vi "drawConnectionArrow.vi"(0 "reference":refnum<class "Graphics.lvclass">, 1 "point2D":T1 {"y" format="%.2f"; "x" format="%.2f"}, 3 "color(if not used=default color)":u32=536870912 format="%.0x", 4 "fill?(F)":bool, 5 "error in (no error)":errorcluster, 6 "Label":string, 8 "Can'tGoLeft":bool) -> (14 "reference out":refnum<class "Graphics.lvclass">, 19 "error out":errorcluster)   [LabVIEW 2016, in "Graphics.lvclass"]
uses:
  <resource>/Framework/Providers/Open_GDS/UML/Graphics_class/Graphics.lvclass
  <resource>/Framework/Providers/Open_GDS/UML/General/Point/Point Point2D.ctl
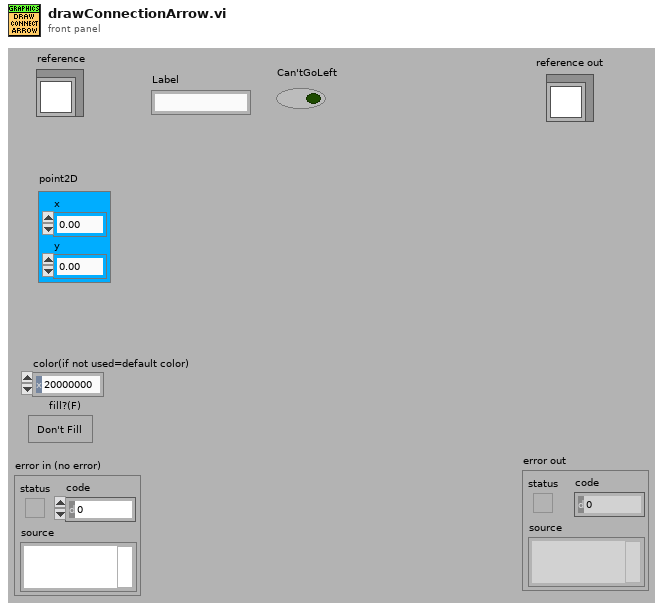
[diagram p1: front panel]
types:
  T1 = typedef "Point Point2D.ctl" = cluster{"x":dbl, "y":dbl}
  T2 = cluster{"horizontal":enum16{"left", "center", "right"}, "vertical":enum16{"top", "center", "bottom"}}
  T3 = typedef "Graphics.lvclass/ObjectAttributes.ctl" = cluster{"drawColor":u32, "backgroundColor":u32, "font":T4, "fontType":T5, "picture":picture, "stroke":T6, "scaleX":dbl, "scaleY":dbl, "screenRef":refnum<vi>, "offsetX":dbl, "offsetY":dbl}
  T4 = typedef "Graphics.lvclass/FontType.ctl" = cluster{"Font Name:":string, "Size":i16, "Strikeout?":bool, "Italic?":bool, "Underline?":bool, "Outline?":bool, "Shadow?":bool, "Bold?":bool}
  T5 = typedef "Graphics.lvclass/LvFontType.ctl" = enum16{"User-specified Font", "Application Font", "System Font", "Dialog Font"}
  T6 = typedef "Graphics.lvclass/StrokeType.ctl" = enum16{"USE_DEFAULT", "SOLID", "DOTTED"}
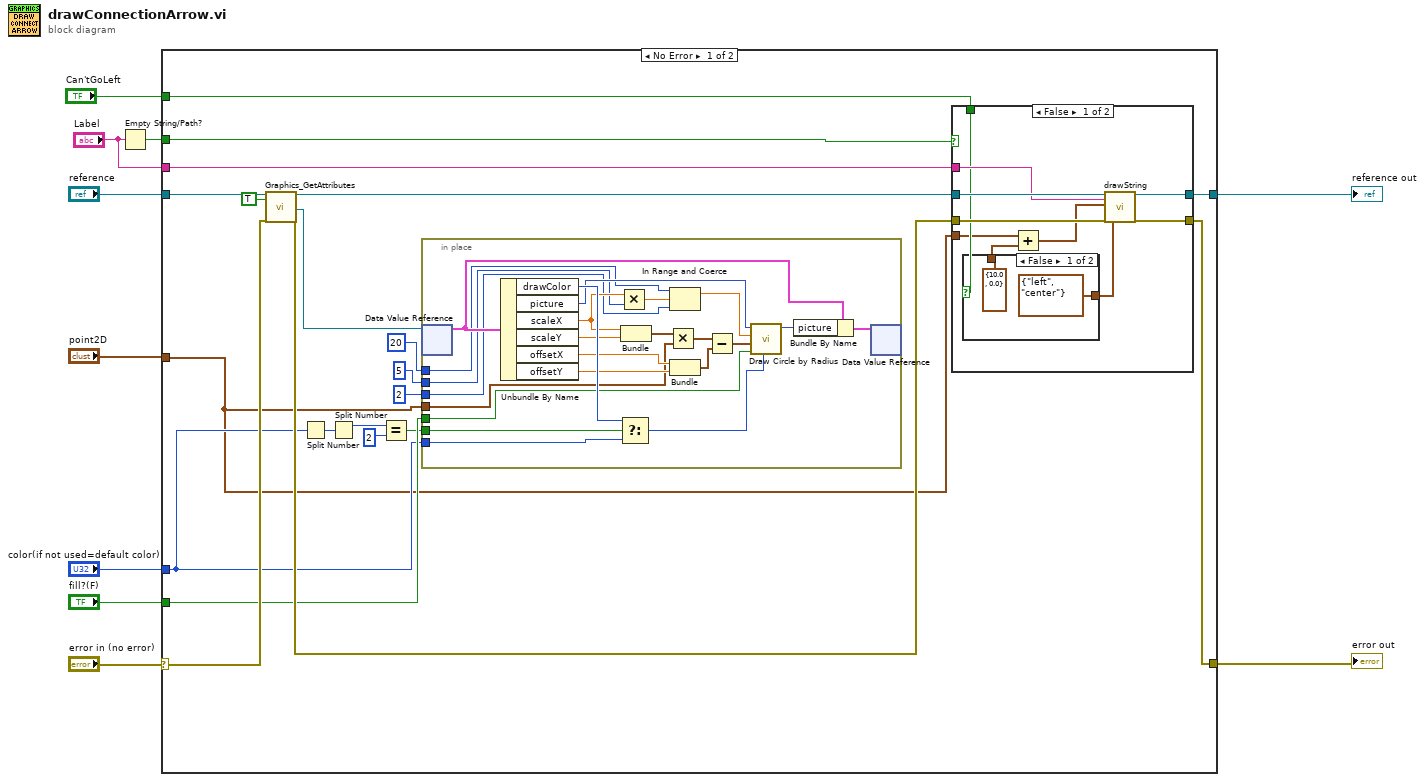
[diagram p0: block diagram]
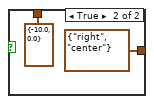
[diagram p2: hidden frame]
diagram:
  n1 = Empty String/Path?(string/path="Label") -> (empty?=w3:bool)
  n2 = case shown="No Error" "error in (no error)" {
    selector: "error in (no error)" -> [w27 w71]
    tunnel: "reference" -> [w31 w72]
    tunnel: [w23 w71] -> w9
    tunnel: [w22 w72] -> w8
    tunnel: "point2D" -> [w11 _]
    tunnel: "color(if not used=default color)" -> [w16 _]
    tunnel: "fill?(F)" -> [w17 _]
    tunnel: w3 -> [w26 _]
    tunnel: "Label" -> [w21 _]
    tunnel: "Can'tGoLeft" -> [w20 _]
    frame No Error {
      n3 = call <resource>:"Graphics_GetAttributes.vi"("reference in"=w31, "OnlyGetDvrReference(False)"=TRUE, "error in (no error)"=w27) -> ("reference out"=w25:refnum<class "Graphics.lvclass">, "DataRef"=w18:refnum<data-value>, "error out"=w24:errorcluster)  [unwired: 13 in, 1 out]
      n4 = Split Number(x=w16) -> (hi(x)=w30:u16)  [unwired: 1 out]
      n5 = Split Number(x=w30) -> (hi(x)=w29:u8)  [unwired: 1 out]
      n6 = Equal?(x=w29, y=u8 2) -> (x = y?=w15:bool)
      n7 = in-place {
        in-place-border: w17 -> [w44]
        in-place-border: w16 -> [w41]
        in-place-border: w15 -> [w40]
        in-place-border: i16 5 ("radius") -> [w38]
        in-place-border: i16 2 ("lower limit") -> [w34]
        in-place-border: i16 20 ("upper limit") -> [w33]
        in-place-border: w11 -> [w32]
        n8 = in-place-dvr #1(w18) -> (w54:T3)  [unwired: 1 out]
        n9 = Unbundle By Name(w54) -> ("drawColor"=w51:u32, "picture"=w50:picture, "scaleX"=w49:dbl, "scaleY"=w48:dbl, "offsetX"=w47:dbl, "offsetY"=w46:dbl)
        n10 = Multiply(x=w49, y=w38) -> (x*y=w37:dbl)
        n11 = Select(t=w51, s=w40, f=w41) -> (s? t:f=w45:u32)
        n12 = Bundle("scaleX"=w49, "scaleY"=w48) -> (w39:cluster{"scaleX":dbl, "scaleY":dbl})  [unwired: 1 out]
        n13 = Multiply(x=w39, y=w32) -> (x*y=w35:T1)
        n14 = In Range and Coerce(upper limit=w33, x=w37, lower limit=w34) -> (coerced(x)=w42:dbl)  [unwired: 1 out]
        n15 = Bundle("offsetX"=w47, "offsetY"=w46) -> (w36:cluster{"offsetX":dbl, "offsetY":dbl})  [unwired: 1 out]
        n16 = Subtract(x=w35, y=w36) -> (x-y=w43:T1)
        n17 = call <vilib>:"Draw Circle by Radius.vi"("color(black)"=w45, "fill?(F)"=w44, "pixel center"=w43, "radius"=w42, "picture"=w50) -> ("new picture"=w53:picture)  [unwired: 3 in, 3 out]
        n18 = Bundle By Name(cluster=w54, "picture"=w53) -> (w52:T3)
        n19 = in-place-dvr #1(w52) -> ()  [unwired: 2 out]
      }
      n20 = case shown="False" w26 {
        tunnel: w25 -> [w64 w70]
        tunnel: w24 -> [w63 w69]
        tunnel: [w62 w69] -> w23
        tunnel: [w61 w70] -> w22
        tunnel: w21 -> [w60 _]
        tunnel: w20 -> [w58 _]
        tunnel: w11 -> [w57 _]
        frame False {
          n21 = case shown="False" w58 {
            tunnel: [T2 {"horizontal"=enum."left", "vertical"=enum."center"} ("alignment(left, top)") T2 {"horizontal"=enum."right", "vertical"=enum."center"} ("alignment(left, top)")] -> w59
            tunnel: [T1 {"x"=10.0, "y"=0.0} ("y") T1 {"x"=-10.0, "y"=0.0} ("y")] -> w55
            frame False {
            }
            frame True {
            }
          }
          n22 = Add(x=w57, y=w55) -> (x+y=w56:T1)
          n23 = call-dynamic "drawString.vi"("reference"=w64, "text"=w60, "textPos"=w56, "error in (no error)"=w63, "alignment(left, top)"=w59) -> ("reference out"=w61:refnum<class "Graphics.lvclass">, "error out"=w62:errorcluster)  [unwired: 2 in, 11 out]
        }
        frame True {
        }
      }
    }
    frame Error {
    }
  }
  "reference out" <- w8
  "error out" <- w9
